vi "APU + 2 Data Replay.vi"() -> ()   [LabVIEW 2015]
uses:
  IP Source/Analog Replay/Settings.ctl
  IP Source/Analog Replay/Input.ctl
  IP Source/Analog Replay/Load Input.ctl
  IP Source/APU/Settings.ctl
  IP Source/APU/Input.ctl
  IP Source/APU/Output.ctl
  IP Source/Version Token.ctl
  IP Source/APU/Shared Settings.ctl
  <vilib>/Platform/TimedLoop/XDataNode/timing_clust.ctl
  <vilib>/Platform/TimedLoop/XDataNode/nitl_modes.ctl
  <vilib>/Platform/TimedLoop/XDataNode/wakeup.ctl
  <vilib>/rvi/Emulation/niFpgaGetClockAttributes.vi
  <vilib>/rvi/Emulation/niFpgaSctlEmulationGetInTimedLoop.vi
  <vilib>/rvi/Emulation/niFpgaEmulationReportErrorSimple.vi
  <vilib>/rvi/DataTransferAndStorage/Container/Common/niFpgaContainerGetUniqueNameForEmu.vi
  <vilib>/rvi/DataTransferAndStorage/Container/Common/niFpgaContainerSetEmuInfo.vi
  <vilib>/rvi/eio/common/nirviEmuReportErrorAndStop.vi
  <vilib>/rvi/Emulation/niFpgaCriticalErrorInLSC.vi
  <vilib>/rvi/eio/common/nirviEmuTemplateMethod_errors.vi
  <vilib>/rvi/LocalResourceManager/LocalResourceManager.xnode
  <vilib>/Platform/TimedLoop/XDataNode/XDataNode.xnode
  <vilib>/eio/EIONode/EIONode.xnode
  <vilib>/Platform/TimedLoop/XDataNode/XDNodeRunTimeDep.lvlib
  IP Source/Analog Replay/Analog Replay.lvlib
  IP Source/APU/APU.lvlib
  IP Source/Engine Simulation Toolkit.lvlib
panel:
  in  "go.my apu":bool
  in  "shared settings.my apu":T1 {"start" format="%#.15g"}
  in  "est.version":T2
  out "output.my apu":T3 caption="output"
  in  "input.my apu":T4={"desired speed"=0.0, "reset"=TRUE} caption="input"
  in  "settings.my apu":T5 caption="settings"
  in  "load input.my other replay":T6={"Data"=[0, 0, 0, 0, 0, 0, 0, 0, 0, 0, 0, 0, 0, 0, 0, 0], "LoadOffset"=0, "Done"=FALSE} caption="input"
  in  "load input.my replay":T6={"Data"=[0, 0, 0, 0, 0, 0, 0, 0, 0, 0, 0, 0, 0, 0, 0, 0], "LoadOffset"=0, "Done"=FALSE} caption="input"
  in  "input.my other replay":T7 caption="input"
  in  "settings.my other replay":T8 caption="settings"
  in  "input.my replay":T7 caption="input"
  in  "settings.my replay":T8 caption="settings"
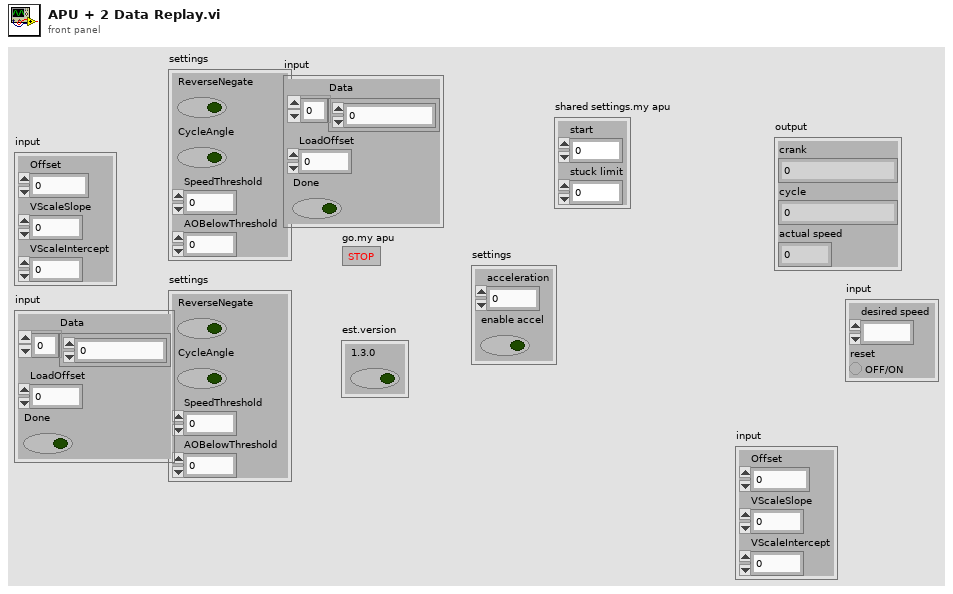
[diagram p1: front panel]
types:
  T1 = typedef "Engine Simulation Toolkit.lvlib/APU.lvlib/Shared Settings.ctl" = cluster{"start":fxp<+,17,17>, "stuck limit":fxp<+,18,18>}
  T2 = typedef "Engine Simulation Toolkit.lvlib/Version Token.ctl" = cluster{"1.3.0":bool}
  T3 = typedef "Engine Simulation Toolkit.lvlib/APU.lvlib/Output.ctl" = cluster{"crank":u16, "cycle":u16, "actual speed":fxp<+/-,23,2>}
  T4 = typedef "Engine Simulation Toolkit.lvlib/APU.lvlib/Input.ctl" = cluster{"desired speed":fxp<+/-,23,2>, "reset":bool}
  T5 = typedef "Engine Simulation Toolkit.lvlib/APU.lvlib/Settings.ctl" = cluster{"acceleration":fxp<+,18,-20>, "enable accel":bool}
  T6 = typedef "Engine Simulation Toolkit.lvlib/Analog Replay.lvlib/Load Input.ctl" = cluster{"Data":i16[], "LoadOffset":u16, "Done":bool}
  T7 = typedef "Engine Simulation Toolkit.lvlib/Analog Replay.lvlib/Input.ctl" = cluster{"Offset":i16, "VScaleSlope":fxp<+,18,6>, "VScaleIntercept":fxp<+/-,18,3>}
  T8 = typedef "Engine Simulation Toolkit.lvlib/Analog Replay.lvlib/Settings.ctl" = cluster{"ReverseNegate":bool, "CycleAngle":bool, "SpeedThreshold":fxp<+/-,23,2>, "AOBelowThreshold":i16}
  T9 = typedef "XDNodeRunTimeDep.lvlib/timing_clust.ctl" = cluster{"Expected End [f-1]":u64, "Actual End [f-1]":u64, "Finished Late? [f-1]":bool, "Expected End [i-1]":u64, "Actual End [i-1]":u64, "Finished Late? [i-1]":bool, "Expected Start [i]":u64, "Actual Start [i]":u64, "Expected Start [f]":u64, "Actual Start [f]":u64, "Source Name":string, "Structure Name":string, "Period":i64, "Deadline":i64, "Offset":i64, "Start":i64, "Priority":i32, "Timeout":i32, "Mode":T10, "Wakeup Reason":T11, "Error":errorcluster, "Source Type":string, "Secondary Source Type":string, "Global End Time":u64, "Global Start Time":u64, "Frame Duration":u64, "Iteration Duration":u64, "Assigned CPU":i32, "I/O Scan Engine Mode":u32}
  T10 = typedef "XDNodeRunTimeDep.lvlib/nitl_modes.ctl" = enum32{"No Change", "Process missed periods, maintain original phase", "Discard missed periods, maintain original phase", "Process missed periods, ignore original phase", "Discard missed periods, ignore original phase"}
  T11 = typedef "XDNodeRunTimeDep.lvlib/wakeup.ctl" = enum32{"Normal", "Aborted", "Asynchronous wakeup", "Timing source error", "Timed loop error", "Timeout"}
  T12 = typedef "Engine Simulation Toolkit.lvlib/APU.lvlib/Register Bus.ctl" = cluster{"Speed":refnum<k21>, "Crank Angle":refnum<k21>, "Cycle Angle":refnum<k21>, "Crank Count":refnum<k21>, "Cycle Count":refnum<k21>, "1.25 MHz Counter":refnum<k21>, "Crank Rollover":refnum<k21>, "Cycle Rollover":refnum<k21>, "shared settings":T1}
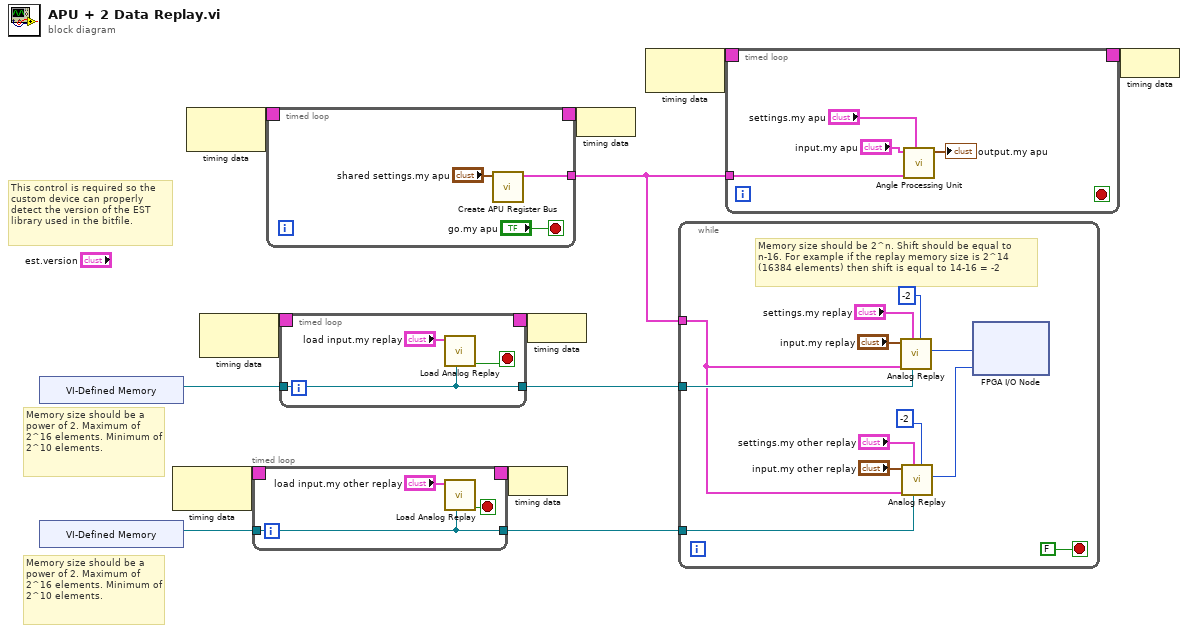
[diagram p0: block diagram]
diagram:
  # "Memory size should be a power of 2. Maximum of 2^16 elements. Minimum of 2^10 elements."
  # "Memory size should be a power of 2. Maximum of 2^16 elements. Minimum of 2^10 elements."
  # "This control is required so the custom device can properly detect the version of the EST library used in the bitfile."
  n1 = xnode "VI-Defined Memory"() -> ("Memory Out"=w12:refnum<k21>)
  n2 = xnode "VI-Defined Memory"() -> ("Memory Out"=w13:refnum<k21>)
  n3 = node-c288() -> (w8:T9)  [unwired: 1 in]
  n4 = node-c288() -> (w2:T9)  [unwired: 1 in]
  n5 = node-c288() -> (w11:T9)  [unwired: 1 in]
  n6 = timed-loop {
    timing: w8 -> [_]
    timing-out: [_] -> w7
    tunnel: w13 -> [w14]
    tunnel: [w14] -> w6
    stop <- w15 stop-if-true
    n7 = call "Load Analog Replay.vi"("memory"=w14, "load input.<user name>"="load input.my other replay") -> ("done"=w15:bool)  [unwired: 9 in]
  }
  n8 = timed-loop {
    timing: w2 -> [_]
    timing-out: [_] -> w1
    tunnel: [w21] -> w3
    stop <- "go.my apu" stop-if-true
    n9 = call "Create APU Register Bus.vi"("shared settings.<user name>"="shared settings.my apu") -> ("register bus"=w21:T12)  [unwired: 10 in]
  }
  n10 = timed-loop {
    timing: w11 -> [_]
    timing-out: [_] -> w10
    tunnel: w12 -> [w24]
    tunnel: [w24] -> w9
    stop <- w25 stop-if-true
    n11 = call "Load Analog Replay.vi"("memory"=w24, "load input.<user name>"="load input.my replay") -> ("done"=w25:bool)  [unwired: 9 in]
  }
  n12 = node-c288(w7) -> ()
  n13 = node-c288(w10) -> ()
  n14 = node-c288(w1) -> ()
  n15 = node-c288() -> (w5:T9)  [unwired: 1 in]
  n16 = while {
    tunnel: w9 -> [w40]
    tunnel: w3 -> [w29]
    tunnel: w6 -> [w37]
    stop <- FALSE stop-if-true
    # "Memory size should be 2^n. Shift should be equal to n-16. For example if the replay memory size is 2^14 (16384 elements) then shift is equal to 14-16 = -2"
    n17 = call "Analog Replay.vi"("shift"=i8 -2, "memory"=w40, "settings.<user name>"="settings.my replay", "register bus"=w29, "input.<user name>"="input.my replay") -> ("analog value"=w33:i16)  [unwired: 6 in]
    n18 = call "Analog Replay.vi"("shift"=i8 -2, "memory"=w37, "settings.<user name>"="settings.my other replay", "register bus"=w29, "input.<user name>"="input.my other replay") -> ("analog value"=w32:i16)  [unwired: 6 in]
    n19 = xnode "FPGA I/O Node"("AO0"=w33, "AO1"=w32) -> ()  [unwired: 2 in, 2 out]
  }
  n20 = timed-loop {
    timing: w5 -> [_]
    timing-out: [_] -> w4
    tunnel: w3 -> [w41]
    stop <- _ stop-if-true
    n21 = call "Angle Processing Unit.vi"("settings.<user name>"="settings.my apu", "register bus"=w41, "input.<user name>"="input.my apu") -> ("output.<user name>"=→"output.my apu":T3)  [unwired: 8 in]
  }
  n22 = node-c288(w4) -> ()
